vi "Bass SubviUpdated.vi"(0 "Image Dst Out":T2, 8 "error out":errorcluster) -> (9 "Orange Bass LED":bool, 11 "Red Bass LED":bool, 13 "Green Bass LED":bool, 15 "Yellow Bass LED":bool, 19 "Blue Bass LED":bool, 27 "error out 2":errorcluster)   [LabVIEW 2009]
uses:
  <vilib>/vision/Image Controls.llb/IMAQ Image.ctl
  <vilib>/Analysis/3filter.llb/Filter Passband Type.ctl
  <vilib>/Analysis/3filter.llb/Butterworth Filter (DBL).vi
  <vilib>/Analysis/NI_AALBase.lvlib
  <vilib>/vision/NI_Vision_Development_Module.lvlib
panel:
  in  "Yellow Bass":T1={"Global Rectangle"=[40, 272, 657, 396], "Contours"=[{"ID"=enum."External", "Type"=3, "Coordinates"=[40, 272, 657, 396]}]} {"Contours"."Type" items=["No Selection", "Point", "Line", "Rectangle", "Oval", "Polygon", "Freehand Region", "Annulus", "Unused2", "Unused3", "Broken Line", "Freehand Line", "Rotated Rectangle"]}
  in  "Red Bass":T1={"Global Rectangle"=[40, 272, 657, 396], "Contours"=[{"ID"=enum."External", "Type"=3, "Coordinates"=[40, 272, 657, 396]}]} {"Contours"."Type" items=["No Selection", "Point", "Line", "Rectangle", "Oval", "Polygon", "Freehand Region", "Annulus", "Unused2", "Unused3", "Broken Line", "Freehand Line", "Rotated Rectangle"]}
  in  "Orange Bass":T1={"Global Rectangle"=[40, 272, 657, 396], "Contours"=[{"ID"=enum."External", "Type"=3, "Coordinates"=[40, 272, 657, 396]}]} {"Contours"."Type" items=["No Selection", "Point", "Line", "Rectangle", "Oval", "Polygon", "Freehand Region", "Annulus", "Unused2", "Unused3", "Broken Line", "Freehand Line", "Rotated Rectangle"]}
  in  "Green Bass":T1={"Global Rectangle"=[40, 272, 657, 396], "Contours"=[{"ID"=enum."External", "Type"=3, "Coordinates"=[40, 272, 657, 396]}]} {"Contours"."Type" items=["No Selection", "Point", "Line", "Rectangle", "Oval", "Polygon", "Freehand Region", "Annulus", "Unused2", "Unused3", "Broken Line", "Freehand Line", "Rotated Rectangle"]}
  in  "Blue Bass":T1={"Global Rectangle"=[40, 272, 657, 396], "Contours"=[{"ID"=enum."External", "Type"=3, "Coordinates"=[40, 272, 657, 396]}]} {"Contours"."Type" items=["No Selection", "Point", "Line", "Rectangle", "Oval", "Polygon", "Freehand Region", "Annulus", "Unused2", "Unused3", "Broken Line", "Freehand Line", "Rotated Rectangle"]}
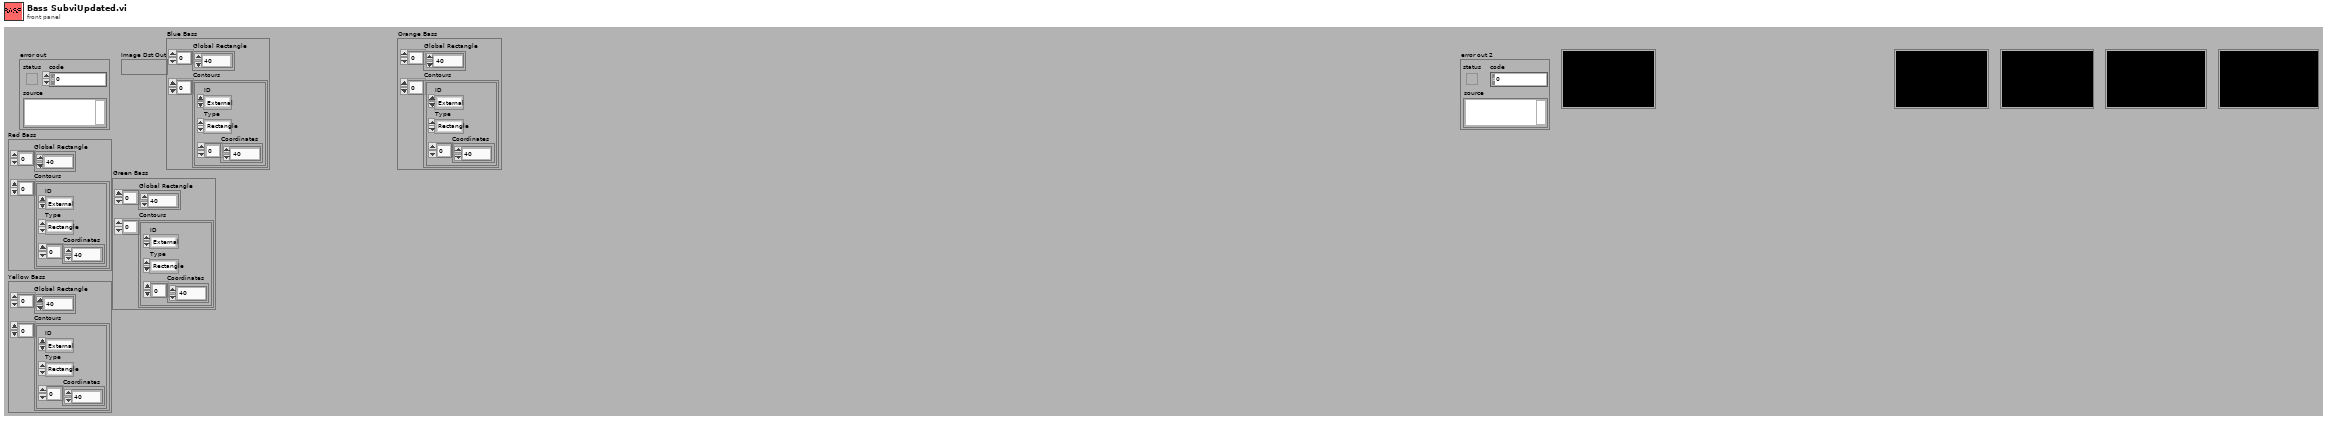
[diagram p1: front panel]
types:
  T1 = cluster{"Global Rectangle":i32[], "Contours":cluster{"ID":enum32{"External", "Internal"}, "Type":u32, "Coordinates":i32[]}[]}
  T2 = typedef "IMAQ Image.ctl" = refnum<image>
  T3 = typedef "NI_AALBase.lvlib/Filter Passband Type.ctl" = enum32{"Lowpass", "Highpass", "Bandpass", "Bandstop"}
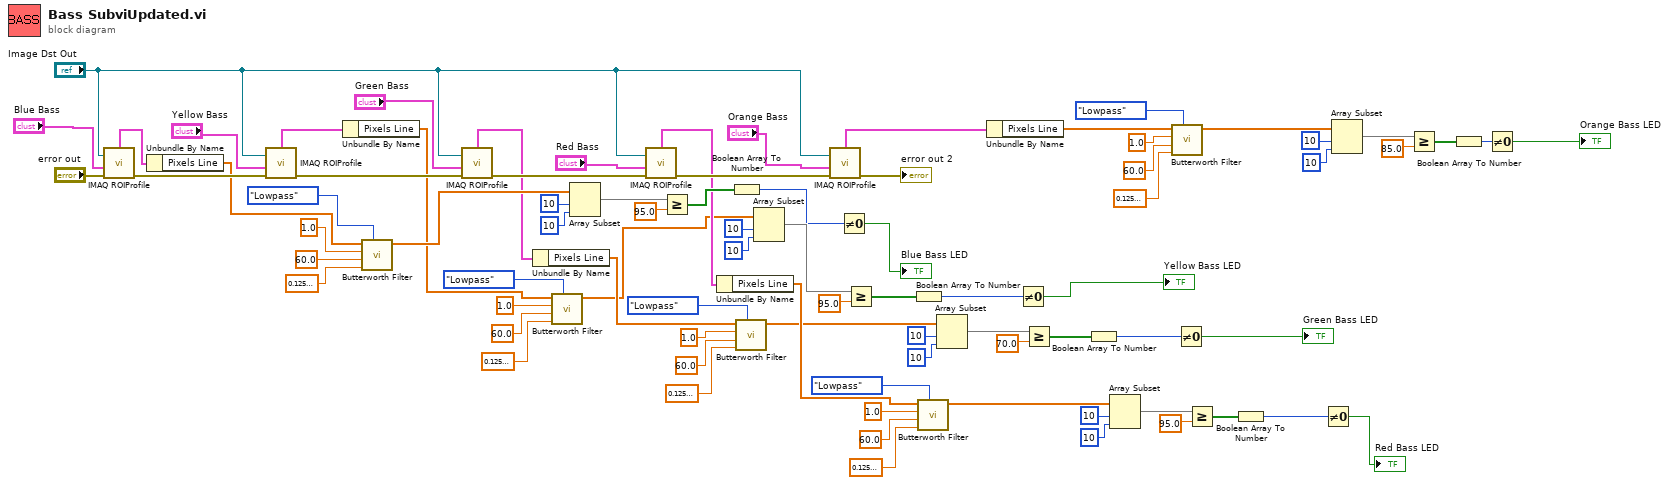
[diagram p0: block diagram]
diagram:
  n1 = call "IMAQ ROIProfile"("error in (no error)"="error out", "ROI Descriptor"="Blue Bass", "Image"="Image Dst Out") -> ("error out"=w29:errorcluster, "ROI Graph"=w30:cluster{"x0":sgl, "dx":sgl, "Pixels Line":sgl[]})  [unwired: 4 out]
  n2 = Unbundle By Name(w30) -> ("Pixels Line"=w7:sgl[])
  n3 = call "IMAQ ROIProfile"("error in (no error)"=w29, "ROI Descriptor"="Yellow Bass", "Image"="Image Dst Out") -> ("error out"=w59:errorcluster, "ROI Graph"=w26:cluster{"x0":sgl, "dx":sgl, "Pixels Line":sgl[]})  [unwired: 4 out]
  n4 = Unbundle By Name(w26) -> ("Pixels Line"=w23:sgl[])
  n5 = call-poly <vilib>:"Butterworth Filter.vi"("filter type"=Filter_Passband_Type."Lowpass", "low cutoff freq: fl"=0.12500000000000006 ("low 2"), "high cutoff freq: fh"=60.0 ("high 8"), "sampling freq: fs"=1.0 ("sampling  8"), "X"=w7) -> ("Filtered X"=w44:dbl[])  [unwired: 3 in, 1 out]
  n6 = call "IMAQ ROIProfile"("error in (no error)"=w59, "ROI Descriptor"="Green Bass", "Image"="Image Dst Out") -> ("error out"=w58:errorcluster, "ROI Graph"=w32:cluster{"x0":sgl, "dx":sgl, "Pixels Line":sgl[]})  [unwired: 4 out]
  n7 = Unbundle By Name(w32) -> ("Pixels Line"=w35:sgl[])
  n8 = call-poly <vilib>:"Butterworth Filter.vi"("filter type"=Filter_Passband_Type."Lowpass", "low cutoff freq: fl"=0.12500000000000006 ("low  7"), "high cutoff freq: fh"=60.0 ("high 7"), "sampling freq: fs"=1.0 ("sampling 7"), "X"=w23) -> ("Filtered X"=w27:dbl[])  [unwired: 3 in, 1 out]
  n9 = Array Subset(array=w44, index=10, length=10) -> (w13:dbl[])
  n10 = call "IMAQ ROIProfile"("error in (no error)"=w58, "ROI Descriptor"="Red Bass", "Image"="Image Dst Out") -> ("error out"=w73:errorcluster, "ROI Graph"=w56:cluster{"x0":sgl, "dx":sgl, "Pixels Line":sgl[]})  [unwired: 4 out]
  n11 = Greater Or Equal?(x=w13, y=95.0) -> (x >= y?=w80:bool[])
  n12 = Unbundle By Name(w56) -> ("Pixels Line"=w53:sgl[])
  n13 = Boolean Array To Number(Boolean array=w80) -> (number=w15:u32)
  n14 = call-poly <vilib>:"Butterworth Filter.vi"("filter type"=Filter_Passband_Type."Lowpass", "low cutoff freq: fl"=0.12500000000000006 ("low  6"), "high cutoff freq: fh"=60.0 ("high 6"), "sampling freq: fs"=1.0 ("sampling 6"), "X"=w35) -> ("Filtered X"=w31:dbl[])  [unwired: 3 in, 1 out]
  n15 = Array Subset(array=w27, index=10, length=10) -> (w18:dbl[])
  n16 = call "IMAQ ROIProfile"("error in (no error)"=w73, "ROI Descriptor"="Orange Bass", "Image"="Image Dst Out") -> ("error out"=→"error out 2":errorcluster, "ROI Graph"=w61:cluster{"x0":sgl, "dx":sgl, "Pixels Line":sgl[]})  [unwired: 4 out]
  n17 = Not Equal To 0?(x=w15) -> (x != 0?=→"Blue Bass LED":bool)
  n18 = Greater Or Equal?(x=w18, y=95.0) -> (x >= y?=w20:bool[])
  n19 = Boolean Array To Number(Boolean array=w20) -> (number=w21:u32)
  n20 = call-poly <vilib>:"Butterworth Filter.vi"("filter type"=Filter_Passband_Type."Lowpass", "low cutoff freq: fl"=0.12500000000000006 ("low  5"), "high cutoff freq: fh"=60.0 ("high 5"), "sampling freq: fs"=1.0 ("sampling 5"), "X"=w53) -> ("Filtered X"=w57:dbl[])  [unwired: 3 in, 1 out]
  n21 = Array Subset(array=w31, index=10, length=10) -> (w40:dbl[])
  n22 = Unbundle By Name(w61) -> ("Pixels Line"=w64:sgl[])
  n23 = Not Equal To 0?(x=w21) -> (x != 0?=→"Yellow Bass LED":bool)
  n24 = Greater Or Equal?(x=w40, y=70.0) -> (x >= y?=w38:bool[])
  n25 = Boolean Array To Number(Boolean array=w38) -> (number=w37:u32)
  n26 = Array Subset(array=w57, index=10, length=10) -> (w48:dbl[])
  n27 = call-poly <vilib>:"Butterworth Filter.vi"("filter type"=Filter_Passband_Type."Lowpass", "low cutoff freq: fl"=0.12500000000000006 ("low  8"), "high cutoff freq: fh"=60.0 ("high 9"), "sampling freq: fs"=1.0 ("sampling 8"), "X"=w64) -> ("Filtered X"=w60:dbl[])  [unwired: 3 in, 1 out]
  n28 = Not Equal To 0?(x=w37) -> (x != 0?=→"Green Bass LED":bool)
  n29 = Greater Or Equal?(x=w48, y=95.0) -> (x >= y?=w50:bool[])
  n30 = Boolean Array To Number(Boolean array=w50) -> (number=w51:u32)
  n31 = Not Equal To 0?(x=w51) -> (x != 0?=→"Red Bass LED":bool)
  n32 = Array Subset(array=w60, index=10, length=10) -> (w69:dbl[])
  n33 = Greater Or Equal?(x=w69, y=85.0) -> (x >= y?=w67:bool[])
  n34 = Boolean Array To Number(Boolean array=w67) -> (number=w66:u32)
  n35 = Not Equal To 0?(x=w66) -> (x != 0?=→"Orange Bass LED":bool)
